vi "APC_9056_SetPathsTS.vi"() -> (0 "Full disk":bool, 1 "No disk":bool=TRUE, 2 "TS signals path":string)   [LabVIEW 2020]
panel:
  out "free disk":dbl
  out "Saving path":string="/u/"
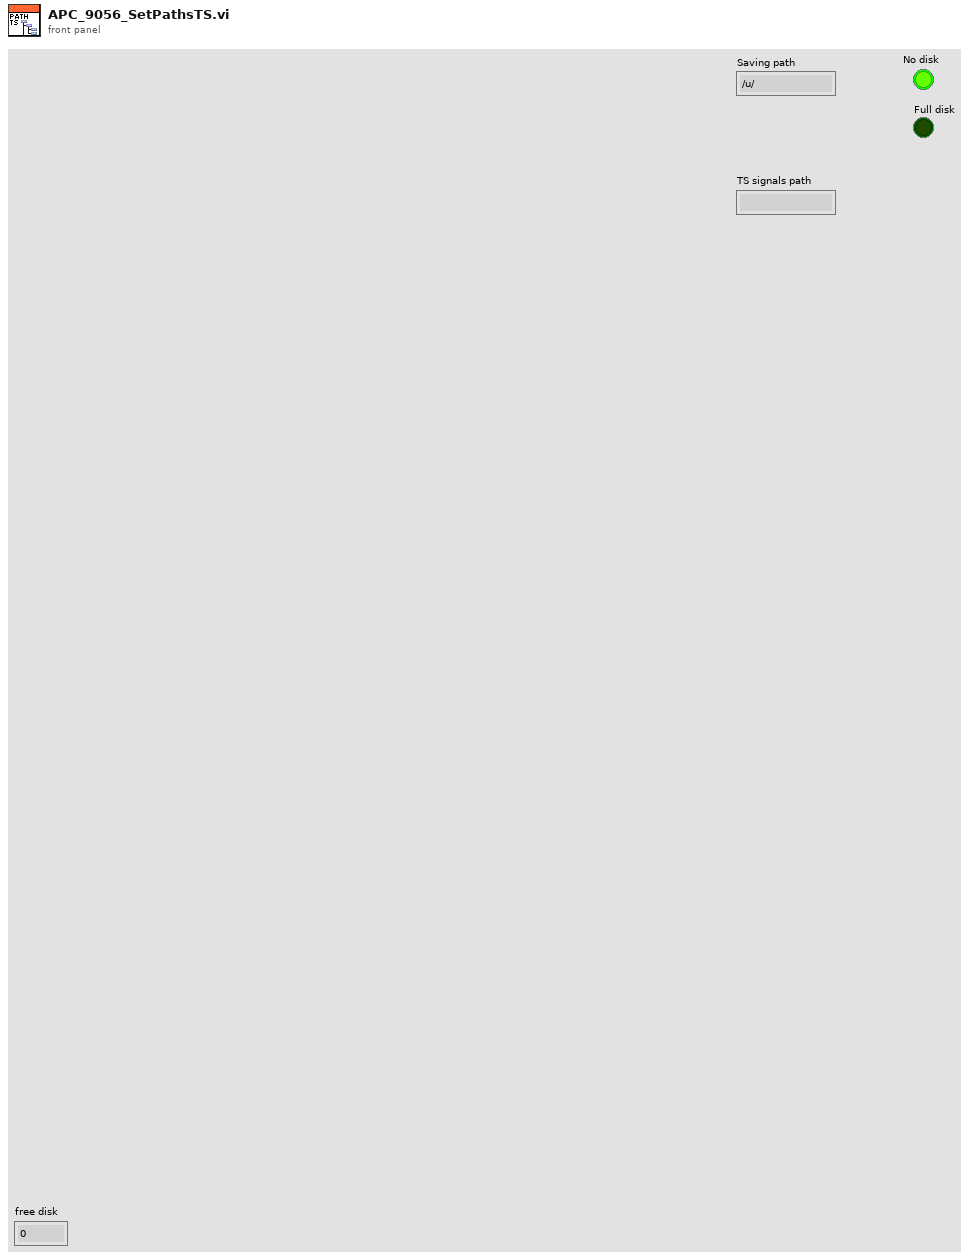
[diagram p1: front panel]
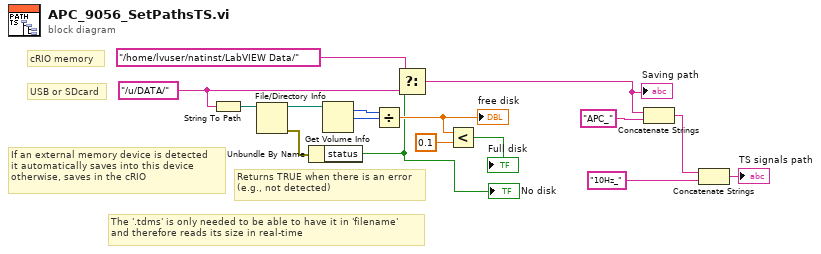
[diagram p0: block diagram]
diagram:
  w2 = "/u/DATA/"
  # "If an external memory device is detected\nit automatically saves into this device\notherwise, saves in the cRIO"
  # "Returns TRUE when there is an error\n(e.g., not detected)"
  # "cRIO memory"
  # "USB or SDcard"
  # "The '.tdms' is only needed to be able to have it in 'filename'\nand therefore reads its size in real-time"
  n1 = String To Path(string=w2) -> (path=w13:path)
  n2 = File/Directory Info(path=w13) -> (path out=w11:path, error out=w12:errorcluster)  [unwired: 1 in, 5 out]
  n3 = Unbundle By Name(w12) -> ("status"=w4:bool)
  "No disk" <- w4
  n4 = Get Volume Info(11:w11) -> (1:w9:i64, 2:w10:i64)  [unwired: 1 in, 4 out]
  n5 = Divide(x=w9, y=w10) -> (x/y=w8:dbl)
  "free disk" <- w8
  n6 = Select(t="/home/lvuser/natinst/LabVIEW Data/", s=w4, f=w2) -> (s? t:f=w1:string)
  "Saving path" <- w1
  n7 = Less?(x=w8, y=0.1) -> (x < y?=→"Full disk":bool)
  n8 = Concatenate Strings(w1, "APC_") -> (w15:string)
  n9 = Concatenate Strings(w15, "10Hz_") -> (→"TS signals path":string)
